vi "arraypath.vi"(1 "Array In":path[](array[path]), 2 "Path To Append":path) -> (0 "Array Out":path[](array[path]))   [LabVIEW 2011]
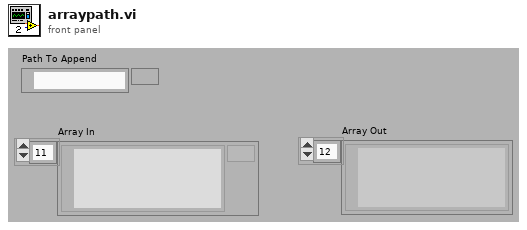
[diagram p1: front panel]
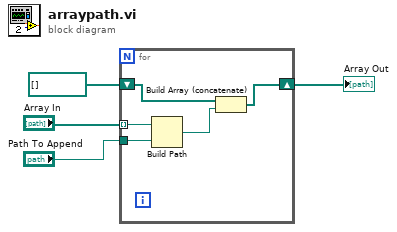
[diagram p0: block diagram]
diagram:
  n1 = for {
    tunnel: "Array In" -> [w6] mode=indexing
    shift-right: [w8] -> w2
    shift-left: path[] [] -> [w9]
    tunnel: "Path To Append" -> [w5]
    n2 = Build Path(base path=w6, name or relative path=w5) -> (appended path=w7:path)
    n3 = Build Array (concatenate)(w9, w7) -> (w8:path[])
  }
  "Array Out" <- w2
